vi "runtest parse step QM.vi"(5 "Step Test ID":string, 7 "Step Number":i32, 9 "Sequence QM allowed?":bool, 11 "POST (empty)":T1) -> (1 "Quickmode?":bool)   [LabVIEW 2011]
uses:
  Addons/internet/utils/keyedarr.llb/Keyed Array.ctl
  Addons/internet/utils/strutil.llb/Case Matching.ctl
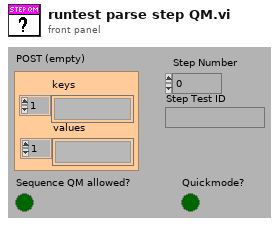
[diagram p1: front panel]
types:
  T1 = typedef "Keyed Array.ctl" = cluster{"keys":string[], "values":string[]}
  T2 = typedef "Case Matching.ctl" = enum16{"a != A", "a == A", "system"}
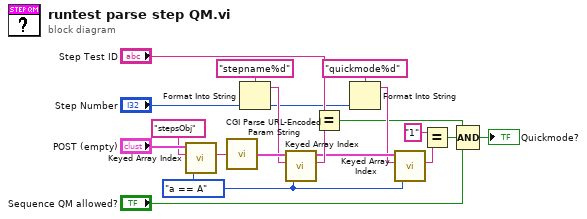
[diagram p0: block diagram]
diagram:
  w5 = Case_Matching."a == A" ("case matching (sensitive)")
  n1 = call "Keyed Array Index.vi"("case matching (sensitive)"=w5, "key"="stepsObj", "array in"="POST (empty)") -> ("value"=w17:string)  [unwired: 1 in, 3 out]
  n2 = call "CGI Parse URL-Encoded Param String.vi"("url-encoded param string"=w17) -> ("params"=w15:T1)
  n3 = Format Into String(format string="stepname%d" ("key"), "Step Number") -> (resulting string=w14:string)  [unwired: 2 in, 1 out]
  n4 = call "Keyed Array Index.vi"("case matching (sensitive)"=w5, "key"=w14, "array in"=w15) -> ("value"=w12:string, "duplicate array"=w11:T1)  [unwired: 1 in, 2 out]
  n5 = Equal?(x="Step Test ID", y=w12) -> (x = y?=w2:bool)
  n6 = Format Into String(format string="quickmode%d" ("key"), "Step Number") -> (resulting string=w9:string)  [unwired: 2 in, 1 out]
  n7 = call "Keyed Array Index.vi"("case matching (sensitive)"=w5, "key"=w9, "array in"=w11) -> ("value"=w7:string)  [unwired: 1 in, 3 out]
  n8 = Equal?(x="1", y=w7) -> (x = y?=w3:bool)
  n9 = Compound Arithmetic op=AND(w2, w3, "Sequence QM allowed?") -> (→"Quickmode?":bool)
